vi "Initialize.vi"(7 "Timeout (30000)":u32=30000, 8 "error in (no error)":errorcluster, 9 "Reset? (T: Yes)":bool=TRUE, 10 "ID Query? (T: Yes)":bool=TRUE, 11 "VISA resource name":refnum<visa-resource-name>="Ceyear") -> (0 "error out":errorcluster, 3 "VISA resource name out":refnum<visa-resource-name>)   [LabVIEW 2021, in "Ceyear.lvlib"]
doc: "Establishes communication with the instrument and optionally performs an instrument identification query and/or an instrument reset. It also places the instrument in a default state needed for other instrument driver operations. Therefore, call this VI before calling other instrument driver VIs for this instrument. Generally, you need to call the <b>Initialize</b> VI only once at the beginning of an application."
uses:
  <instrlib>/Ceyear/Ceyear.lvlib
panel:
  in  "Password (empty)":string
  in  "User Name (anonymous)":string="anonymous"
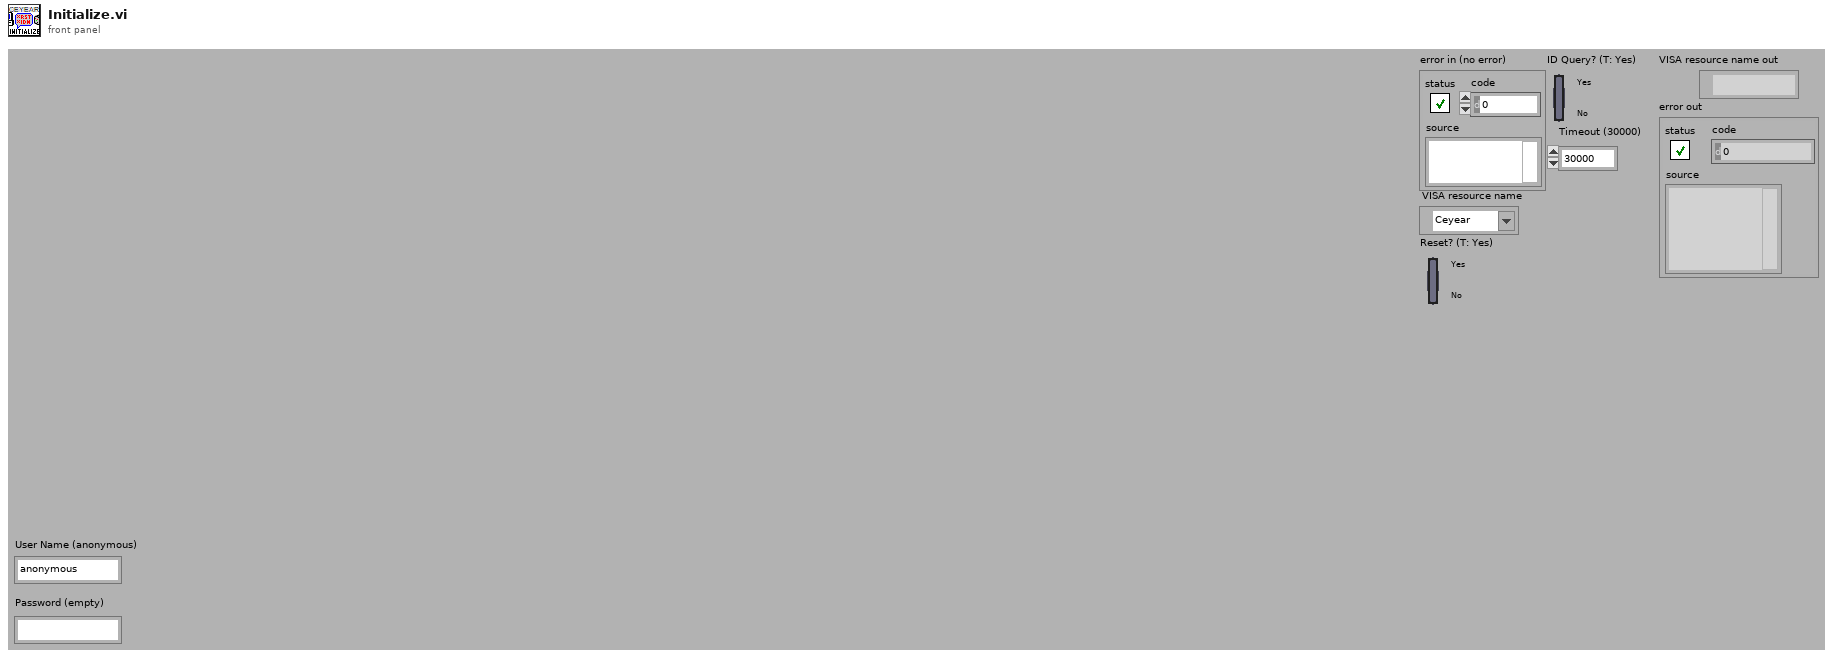
[diagram p1: front panel]
types:
  T1 = cluster{"status":bool, "code":i32, "VI name":string}
  T2 = cluster{"Status":bool, "Code":i32, "Source (VI Name)":string}
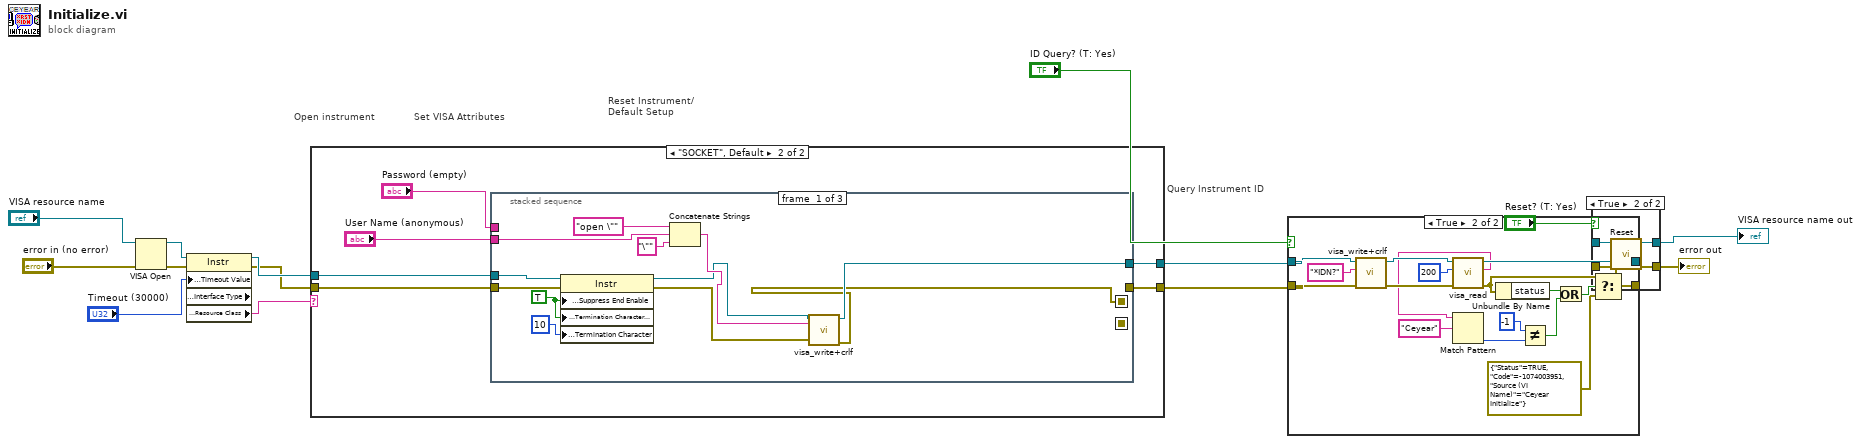
[diagram p0: block diagram]
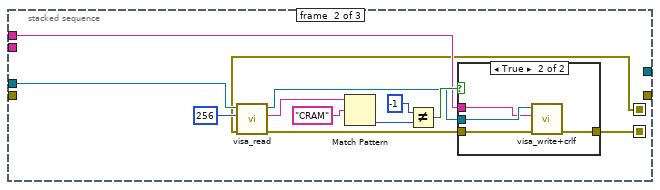
[diagram p4: hidden frame]
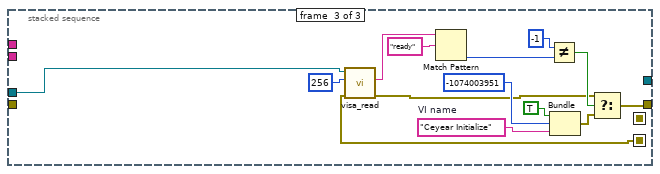
[diagram p6: hidden frame]
diagram:
  # "Set VISA Attributes"
  # "Query Instrument ID"
  # "Reset Instrument/\nDefault Setup"
  # "Open instrument"
  n1 = VISA Open(error in (no error)="error in (no error)", VISA resource name="VISA resource name") -> (VISA resource name=w13:refnum<visa-resource-name>, error out=w11:errorcluster)  [unwired: 3 in]
  n2 = property class="Instr" props=["General Settings:Timeout Value", "Interface Information:Interface Type", "General Settings:Resource Class"](reference=w13, error in=w11, "General Settings:Timeout Value"="Timeout (30000)") -> (reference out=w8:refnum<visa-resource-name>, error out=w7:errorcluster, "General Settings:Resource Class"=w1:string)  [unwired: 1 out]
  n3 = case shown="\"SOCKET\", Default" w1 {
    tunnel: w8 -> [w18 w24]
    tunnel: w7 -> [w17 w23]
    tunnel: [w18 w22] -> w6
    tunnel: [w17 w21] -> w5
    frame "INSTR" {
    }
    frame "SOCKET", Default {
      n4 = stacked-sequence {
        seq-local: [w25 _ _] -> [_ w37 _]
        seq-local: [_ w44 _] -> [_ _ w56]
        tunnel: w24 -> [w33 w41 w57]
        tunnel: w23 -> [w32 _ _]
        tunnel: [w26 _ _] -> w22
        tunnel: [_ _ w64] -> w21
        tunnel: "User Name (anonymous)" -> [w36 _ _]
        tunnel: "Password (empty)" -> [_ w43 _]
        frame #0 {
          w31 = TRUE items=["OFF", "ON", "OFF", "ON"]
          n5 = property class="Instr"(reference=w33, error in=w32, "Message Based Settings:Suppress End Enable"=w31, "Message Based Settings:Termination Character Enable"=w31, "Message Based Settings:Termination Character"=u8 10) -> (reference out=w28:refnum<visa-resource-name>, error out=w27:errorcluster)
          n6 = Concatenate Strings("open \"", w36, "\"") -> (w29:string)
          n7 = call <instrlib>:"visa_write+crlf.vi"("error in (no error)"=w27, "Strings (empty)"=w29, "VISA resource name"=w28) -> ("error out"=w25:errorcluster, "VISA resource name out"=w26:refnum<visa-resource-name>)  [unwired: 7 in]
        }
        frame #1 {
          n8 = call <instrlib>:"visa_read.vi"("error in (no error)"=w37, "Byte Count (0)"=u32 256, "VISA resource name"=w41) -> ("error out"=w38:errorcluster, "Read Data"=w39:string, "VISA resource name out"=w40:refnum<visa-resource-name>)  [unwired: 5 in, 1 out]
          n9 = Match Pattern(string=w39, regular expression="CRAM") -> (offset past match=w47:i32)  [unwired: 1 in, 3 out]
          n10 = Not Equal?(x=-1, y=w47) -> (x != y?=w45:bool)
          n11 = case shown="True" w45 {
            tunnel: [w49 w50] -> w44
            tunnel: w40 -> [_ w52]
            tunnel: w38 -> [w49 w53]
            tunnel: w43 -> [_ w51]
            frame False {
            }
            frame True {
              n12 = call <instrlib>:"visa_write+crlf.vi"("error in (no error)"=w53, "Strings (empty)"=w51, "VISA resource name"=w52) -> ("error out"=w50:errorcluster)  [unwired: 7 in, 1 out]
            }
          }
        }
        frame #2 {
          w61 = "Ceyear Initialize"  # VI name
          n13 = call <instrlib>:"visa_read.vi"("error in (no error)"=w56, "Byte Count (0)"=u32 256, "VISA resource name"=w57) -> ("error out"=w55:errorcluster, "Read Data"=w54:string)  [unwired: 5 in, 2 out]
          n14 = Match Pattern(string=w54, regular expression="ready") -> (offset past match=w66:i32)  [unwired: 1 in, 3 out]
          n15 = Not Equal?(x=-1, y=w66) -> (x != y?=w63:bool)
          n16 = Bundle(TRUE, -1074003951, "VI name"=w61) -> (w59:cluster{bool, i32, "VI name":string})  [unwired: 1 in]
          n17 = Select(t=w55, s=w63, f=w59) -> (s? t:f=w64:T1)
        }
      }
    }
  }
  n18 = case shown="True" "ID Query? (T: Yes)" {
    tunnel: [w68 w86] -> w2
    tunnel: [w69 w75] -> w3
    tunnel: w6 -> [w69 w73]
    tunnel: w5 -> [w68 w72]
    frame False {
    }
    frame True {
      n19 = call <instrlib>:"visa_write+crlf.vi"("error in (no error)"=w72, "Strings (empty)"="*IDN?", "VISA resource name"=w73) -> ("error out"=w77:errorcluster, "VISA resource name out"=w78:refnum<visa-resource-name>)  [unwired: 7 in]
      n20 = call <instrlib>:"visa_read.vi"("error in (no error)"=w77, "Byte Count (0)"=u32 200, "VISA resource name"=w78) -> ("error out"=w74:errorcluster, "Read Data"=w70:string, "VISA resource name out"=w75:refnum<visa-resource-name>)  [unwired: 5 in, 1 out]
      n21 = Match Pattern(string=w70, regular expression="Ceyear") -> (offset past match=w80:i32)  [unwired: 1 in, 3 out]
      n22 = Unbundle By Name(w74) -> ("status"=w83:bool)
      n23 = Not Equal?(x=-1, y=w80) -> (x != y?=w85:bool)
      n24 = Or(x=w83, y=w85) -> (x .or. y?=w84:bool)
      n25 = Select(t=w74, s=w84, f=T2 {"Status"=TRUE, "Code"=-1074003951, "Source (VI Name)"="Ceyear Initialize"}) -> (s? t:f=w86:T2)
    }
  }
  n26 = case shown="True" "Reset? (T: Yes)" {
    tunnel: w2 -> [w87 w89]
    tunnel: [w87 w92] -> w9
    tunnel: w3 -> [w88 w90]
    tunnel: [w88 w91] -> w10
    frame False {
    }
    frame True {
      n27 = call <instrlib>:"Reset.vi"("error in (no error)"=w89, "VISA resource name"=w90) -> ("error out"=w92:errorcluster, "VISA resource name out"=w91:refnum<visa-resource-name>)  [unwired: 8 in]
    }
  }
  "VISA resource name out" <- w10
  "error out" <- w9
